vi "Realtime.vi"() -> ()   [LabVIEW 2011]
uses:
  <vilib>/measure/maspectr.llb/FFT Power Spectrum and PSD for N Chan.vi
  <vilib>/gmath/NI_Gmath.lvlib
  <vilib>/measure/NI_MAPro.lvlib
  <vilib>/ptbypt/NI_PtbyPt.lvlib
panel:
  out "STFT Spectrogram Substraction":dbl[][](graph)
  out "Current  before":dynamicdata(graph)
  out "Current  after":dynamicdata(graph)
  out "Current":cluster{"f0":dbl, "df":dbl, "magnitude":dbl[]}[](graph)
  out "STFT Spectrogram  Current":dbl[][](graph)
  out "light spectrum":cluster{"f0":dbl, "df":dbl, "magnitude":dbl[]}[](graph)
  out "Ligth intensity  after":dynamicdata(graph)
  in  "Cut off frequency":i32=200
  out "STFT Spectrogram Light":dbl[][](graph)
  in  "Sampling Frequency":i32=200
  in  "window info":cluster{"type":u32, "length":i32}={"type"=1, "length"=64} {"type" items=["Rectangle"=0, "Hanning"=1, "Hamming"=2, "Blackman-Harris"=3, "Exact Blackman"=4, "Blackman"=5, "Flat Top"=6, "4 Term B-Harris "=7, "7 Term B-Harris"=8, "Low Sidelobe"=9, "Blackman Nuttall"=11, "Triangle"=30, "Gaussian"=62]}
  in  "time-freq sampling info":cluster{"time steps":i32, "frequency bins":i32}={"time steps"=4, "frequency bins"=512}
  out "Ligth intensity before":dynamicdata(graph)
  out "light history":dynamicdata(graph)
  in  "stop":bool
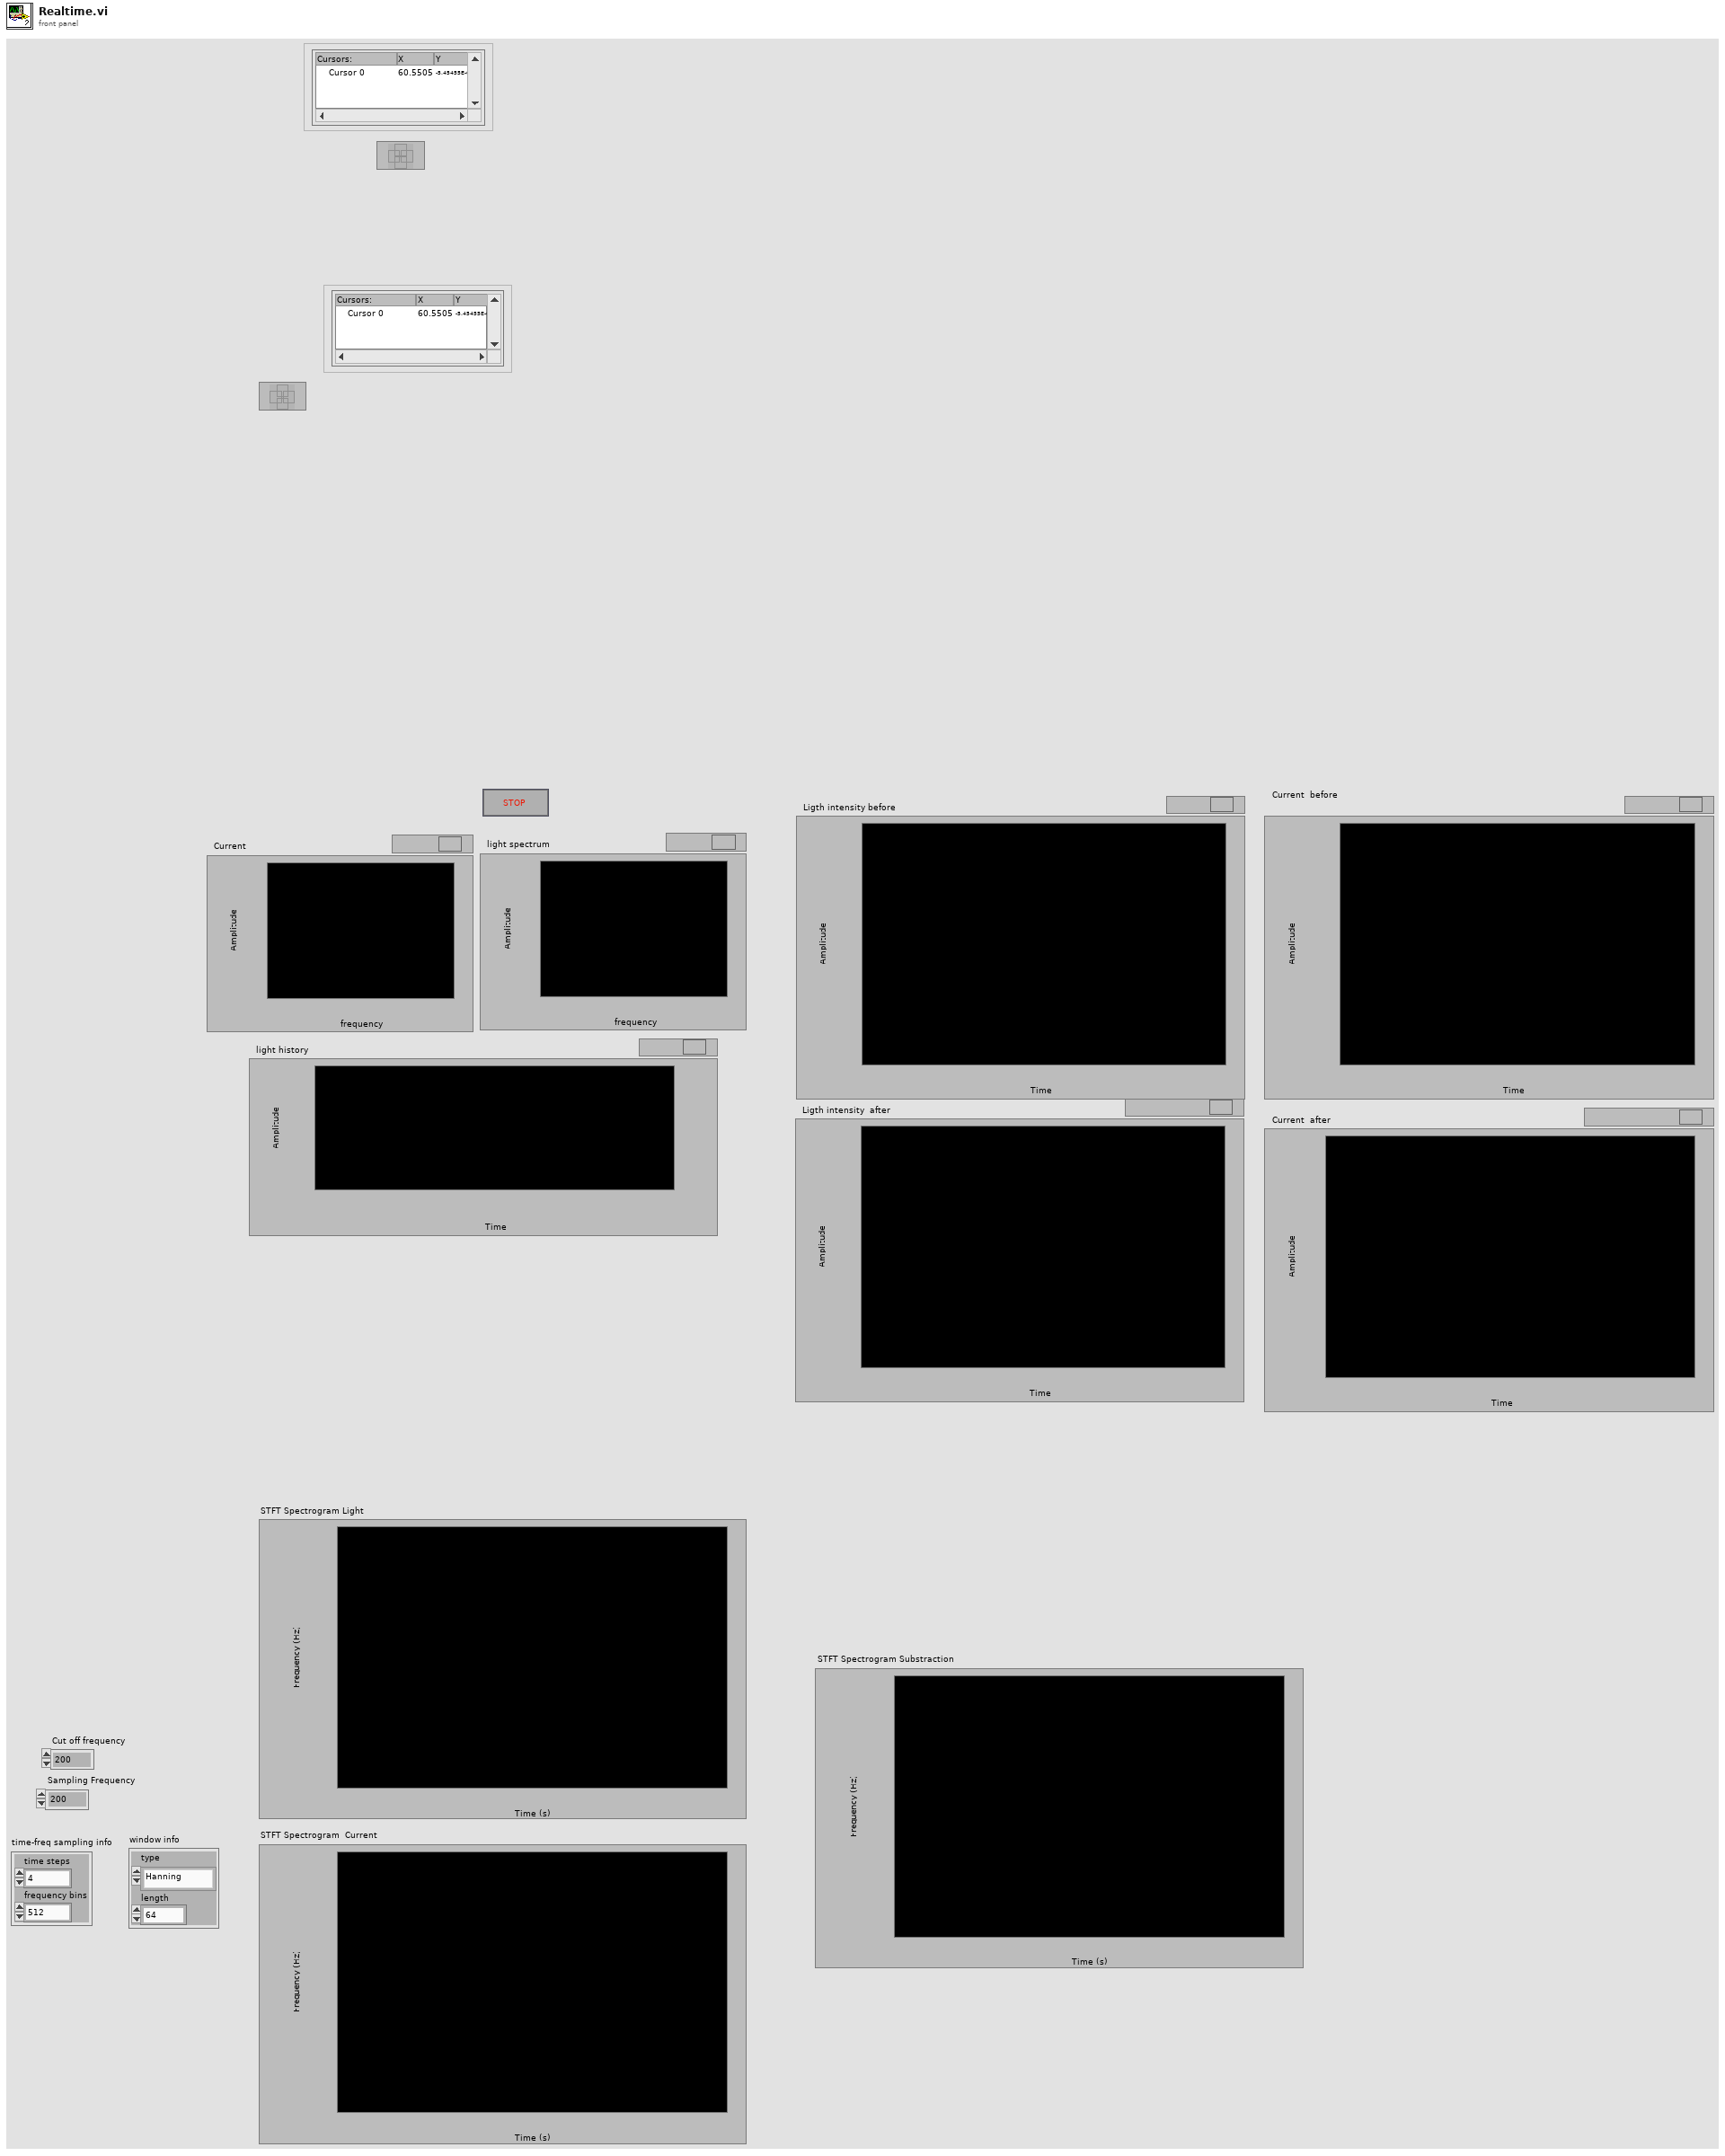
[diagram p1: front panel]
types:
  T1 = enum16{"fire", "rainbow", "grey", "inverse grey", "ice", "original"}
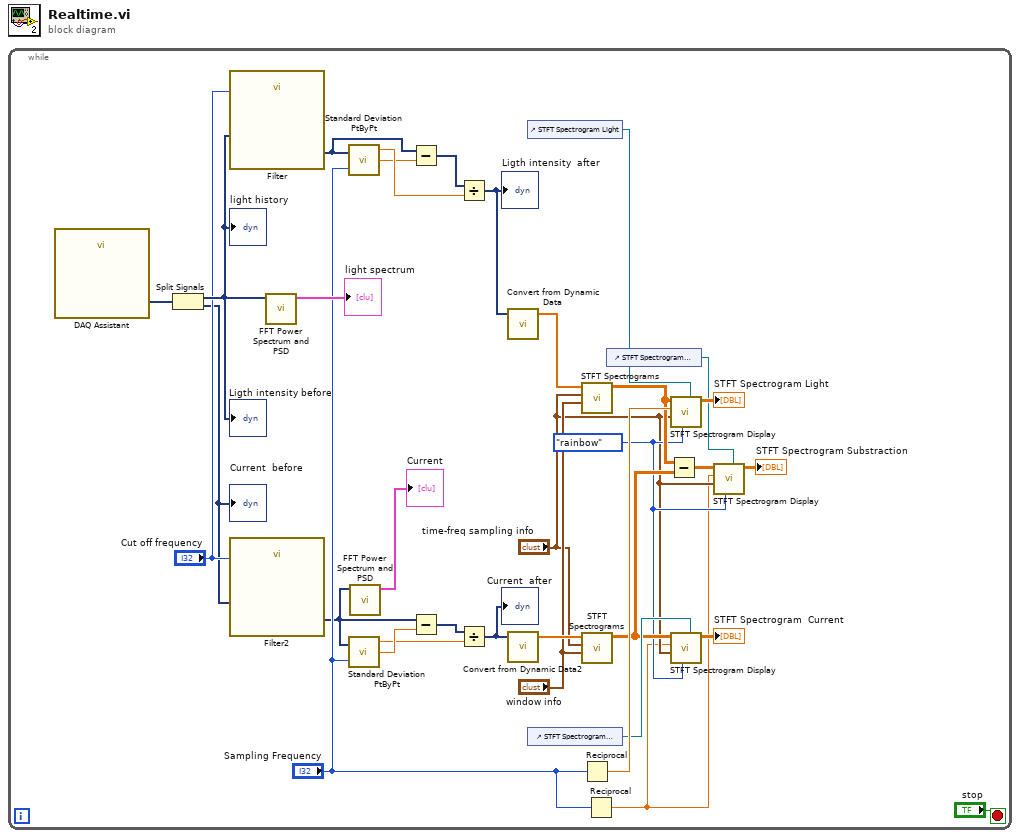
[diagram p0: block diagram]
diagram:
  n1 = while {
    stop <- "stop" stop-if-true
    w7 = T1."rainbow" ("map selector")
    n2 = call "DAQ Assistant"() -> ("data"=w23:dynamicdata)  [unwired: 16 in, 3 out]
    n3 = Split Signals(w23) -> (w22:dynamicdata, w18:dynamicdata)  [unwired: 2 in]
    "light history" <- w22
    "Ligth intensity before" <- w22
    "Current  before" <- w18
    n4 = call "Filter"("Lower Cut-Off"="Cut off frequency", "Signal"=w22) -> ("Filtered Signal"=w17:dynamicdata)  [unwired: 8 in, 1 out]
    n5 = call "Filter2"("Lower Cut-Off"="Cut off frequency", "Signal"=w18) -> ("Filtered Signal"=w15:dynamicdata)  [unwired: 8 in, 1 out]
    n6 = call-poly <vilib>:"FFT Power Spectrum and PSD.vi"("time signals"=w22) -> ("Power Spectrum / PSD"=→"light spectrum":cluster{"f0":dbl, "df":dbl, "magnitude":dbl[]}[])  [unwired: 7 in, 3 out]
    n7 = call <vilib>:"Standard Deviation PtByPt.vi"("x"=w17, "sample length"="Sampling Frequency") -> ("standard deviation"=w4:dbl, "mean"=w3:dbl)  [unwired: 1 in, 1 out]
    n8 = call <vilib>:"Standard Deviation PtByPt.vi"("x"=w15, "sample length"="Sampling Frequency") -> ("standard deviation"=w13:dbl, "mean"=w14:dbl)  [unwired: 1 in, 1 out]
    n9 = call-poly <vilib>:"FFT Power Spectrum and PSD.vi"("time signals"=w15) -> ("Power Spectrum / PSD"=→"Current":cluster{"f0":dbl, "df":dbl, "magnitude":dbl[]}[])  [unwired: 7 in, 3 out]
    n10 = Subtract(x=w17, y=w3) -> (x-y=w20:dynamicdata)
    n11 = Subtract(x=w15, y=w14) -> (x-y=w19:dynamicdata)
    n12 = Divide(x=w20, y=w4) -> (x/y=w2:dynamicdata)
    "Ligth intensity  after" <- w2
    n13 = Divide(x=w19, y=w13) -> (x/y=w1:dynamicdata)
    "Current  after" <- w1
    n14 = call "Convert from Dynamic Data"("Dynamic Data Type"=w2) -> ("Array"=w32:dbl[])  [unwired: 3 in]
    n15 = call "Convert from Dynamic Data2"("Dynamic Data Type"=w1) -> ("Array"=w28:dbl[])  [unwired: 3 in]
    n16 = control-ref of="STFT Spectrogram Light"() -> (w30:refnum<vi>)
    n17 = control-ref of="STFT Spectrogram  Current"() -> (w26:refnum<vi>)
    n18 = call <vilib>:"STFT Spectrograms.vi"("window info"="window info", "time-freq sampling info"="time-freq sampling info", "X"=w32) -> ("STFT Spectrogram {X}"=w12:dbl[][])  [unwired: 3 in, 5 out]
    n19 = call <vilib>:"STFT Spectrograms.vi"("window info"="window info", "time-freq sampling info"="time-freq sampling info", "X"=w28) -> ("STFT Spectrogram {X}"=w11:dbl[][])  [unwired: 3 in, 5 out]
    n20 = Reciprocal(x="Sampling Frequency") -> (1/x=w33:dbl)
    n21 = Reciprocal(x="Sampling Frequency") -> (1/x=w5:dbl)
    n22 = control-ref of="STFT Spectrogram  Substraction"() -> (w8:refnum<vi>)
    n23 = Subtract(x=w12, y=w11) -> (x-y=w10:dbl[][])
    n24 = call "STFT Spectrogram Display.vi"("Intensity Graph"=w30, "map selector"=w7, "time-freq sampling info"="time-freq sampling info", "dt"=w33, "STFT Spectrogram In"=w12) -> ("STFT Spectrogram Out"=→"STFT Spectrogram Light":dbl[][])  [unwired: 1 in, 5 out]
    n25 = call "STFT Spectrogram Display.vi"("Intensity Graph"=w26, "map selector"=w7, "time-freq sampling info"="time-freq sampling info", "dt"=w5, "STFT Spectrogram In"=w11) -> ("STFT Spectrogram Out"=→"STFT Spectrogram  Current":dbl[][])  [unwired: 1 in, 5 out]
    n26 = call "STFT Spectrogram Display.vi"("Intensity Graph"=w8, "map selector"=w7, "time-freq sampling info"="time-freq sampling info", "dt"=w5, "STFT Spectrogram In"=w10) -> ("STFT Spectrogram Out"=→"STFT Spectrogram Substraction":dbl[][])  [unwired: 1 in, 5 out]
  }
